vi "ExplorerTree Example.vi"() -> ()   [LabVIEW 2016]
doc: "This example gets the content of a folder and displays it in a tree control. Similar to file explorer windows, this sorts alphabetically by sub-directories then files. The file extension icons are returned as a custom symbols array to be referenced in the tree control. If a file icon is not found, this queries the operating system shell icon and keeps the glyph cached.\n\nCreated By: Ryan Pacini"
panel:
  in  "Folder Path":path
  in  "Tree":string[](tree)
  # "Instructions: Select folder path then press run"
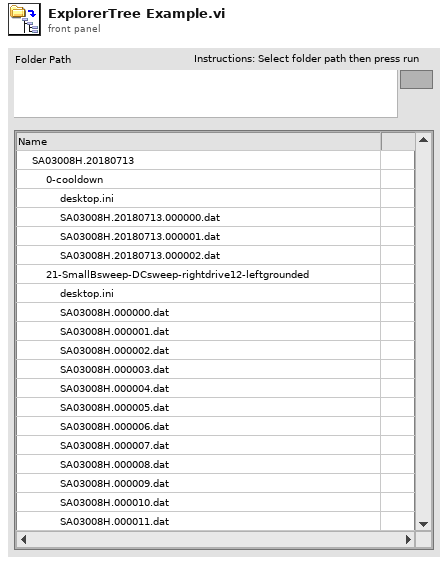
[diagram p1: front panel]
types:
  T1 = typedef "imagedata.ctl" = cluster{"image type":i32, "image depth":i32, "image":u8[], "mask":u8[], "colors":u32[], "Rectangle":cluster{"left":i16, "top":i16, "right":i16, "bottom":i16}}
  T2 = cluster{"Left Cell String":string, "Child Text":string[], "Child Tag":string, "Item Indent":i32, "Child Only?":bool, "Glyph Index":i32}[]
  T3 = cluster{"Left Cell String":string, "Child Text":string[], "Child Tag":string, "Item Indent":i32, "Child Only?":bool, "Glyph Index":i32}
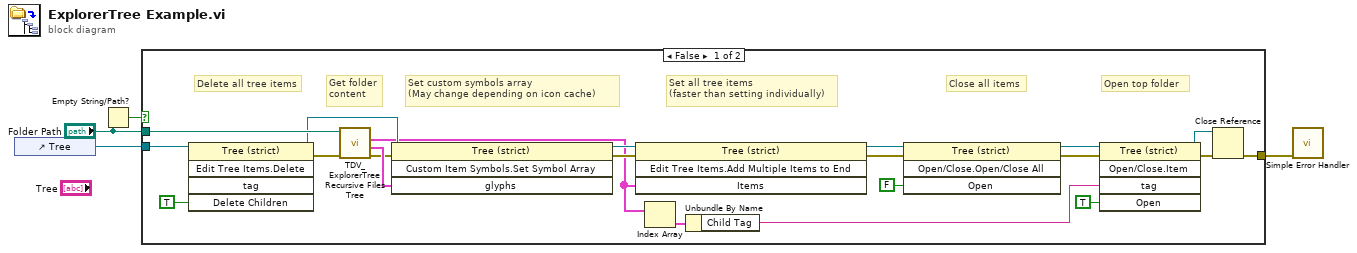
[diagram p0: block diagram]
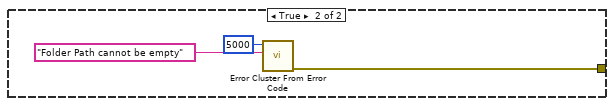
[diagram p2: hidden frame]
diagram:
  n1 = control-ref of="Tree"() -> (w4:refnum<vi>)
  n2 = Empty String/Path?(string/path="Folder Path") -> (empty?=w1:bool)
  n3 = case shown="False" w1 {
    tunnel: w4 -> [w25 _]
    tunnel: "Folder Path" -> [w22 _]
    tunnel: [w6 w26] -> w3
    frame False {
      # "Open top folder"
      # "Close all items"
      # "Set all tree items\n(faster than setting individually)"
      # "Set custom symbols array\n(May change depending on icon cache)"
      # "Get folder\ncontent"
      # "Delete all tree items"
      n4 = invoke class="Tree (strict)" method="Edit Tree Items.Delete"(reference=w25, "Delete Children"=TRUE ("Delete Children?")) -> (reference out=w21:refnum<vi>, error out=w23:errorcluster)  [unwired: 3 in, 3 out]
      n5 = call "TDV_ExplorerTree Recursive Files Tree.vi"("error in (no error)"=w23, "Folder Path"=w22) -> ("error out"=w5:errorcluster, "Glyphs"=w20:T1[], "Items"=w12:T2)  [unwired: 6 in, 1 out]
      n6 = invoke class="Tree (strict)" method="Custom Item Symbols.Set Symbol Array"(reference=w21, error in=w5, "glyphs"=w20) -> (reference out=w18:refnum<vi>, error out=w19:errorcluster)  [unwired: 1 in, 2 out]
      n7 = invoke class="Tree (strict)" method="Edit Tree Items.Add Multiple Items to End"(reference=w18, error in=w19, "Items"=w12) -> (reference out=w16:refnum<vi>, error out=w17:errorcluster)  [unwired: 1 in, 2 out]
      n8 = Index Array(array=w12) -> (element=w11:T3)  [unwired: 1 in]
      n9 = Unbundle By Name(w11) -> ("Child Tag"=w10:string)
      n10 = invoke class="Tree (strict)" method="Open/Close.Open/Close All"(reference=w16, error in=w17, "Open"=FALSE ("Open?")) -> (reference out=w14:refnum<vi>, error out=w13:errorcluster)  [unwired: 1 in, 2 out]
      n11 = invoke class="Tree (strict)" method="Open/Close.Item"(reference=w14, error in=w13, "tag"=w10, "Open"=TRUE ("Open?")) -> (reference out=w7:refnum<vi>, error out=w8:errorcluster)  [unwired: 1 in, 3 out]
      n12 = Close Reference(reference=w7, error in (no error)=w8) -> (error out=w6:errorcluster)
    }
    frame True {
      n13 = call <vilib>:"Error Cluster From Error Code.vi"("error message (\"\")"="Folder Path cannot be empty" ("source"), "error code (0)"=5000) -> ("error out"=w26:errorcluster)  [unwired: 7 in]
    }
  }
  n14 = call <vilib>:"Simple Error Handler.vi"("error in (no error)"=w3) -> ()  [unwired: 4 in, 5 out]
